vi "Launch UI.vi"(8 "error in (no error)":errorcluster, 11 "Test Application Controller in":refnum<class "Test Application Controller.lvclass">) -> (0 "error out":errorcluster, 3 "Test Application Controller out":refnum<class "Test Application Controller.lvclass">)   [LabVIEW 2017, in "Test Application Controller.lvlib" / "Test Application Controller.lvclass"]
uses:
  Test Application Controller.lvclass
  C:/Program Files (x86)/National Instruments/LabVIEW 2017/vi.lib/ActorFramework/Actor/Actor.lvclass
  User Interface/User Interface.lvclass
  Test Application Controller Messages/Start Test Msg/Start Test Msg.lvclass
  D:/Career/Tesla/LabVIEW_Interview_Problem/Tesla Test Application/User Interface Messages/Start Test Msg/Start Test Msg.lvclass
  Test Application Controller Messages/Close Application Msg/Close Application Msg.lvclass
  D:/Career/Tesla/LabVIEW_Interview_Problem/Tesla Test Application/User Interface Messages/Close Application Msg/Close Application Msg.lvclass
  Test Application Controller Messages/Stop Test Msg/Stop Test Msg.lvclass
  D:/Career/Tesla/LabVIEW_Interview_Problem/Tesla Test Application/User Interface Messages/Stop Test Msg/Stop Test Msg.lvclass
  Test Application Controller Messages/Generate Report Msg/Generate Report Msg.lvclass
  D:/Career/Tesla/LabVIEW_Interview_Problem/Tesla Test Application/User Interface Messages/Generate Report Msg/Generate Report Msg.lvclass
  User Interface/User Interface.lvclass/User Interface.ctl
  Test Application Controller.lvclass/Test Application Controller.ctl
  <vilib>/ActorFramework/Actor/Actor.lvclass
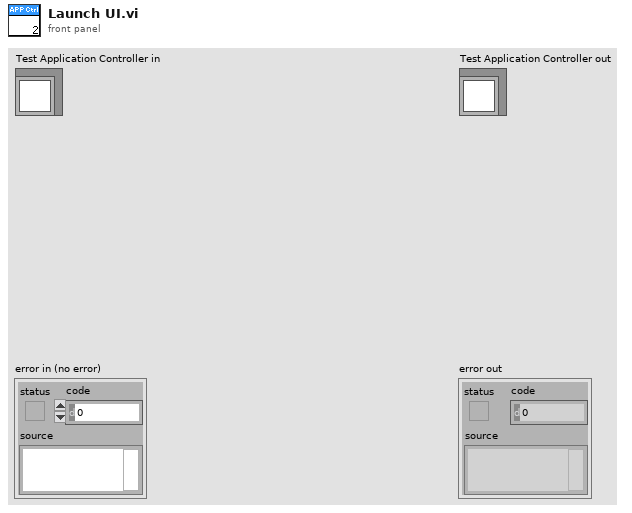
[diagram p1: front panel]
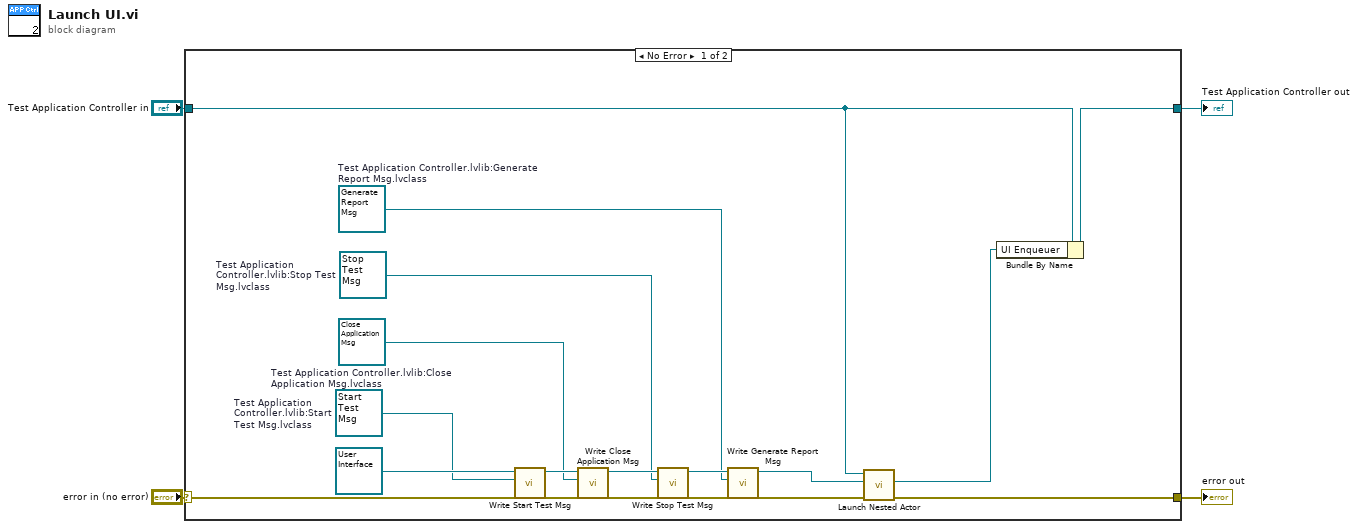
[diagram p0: block diagram]
diagram:
  n1 = case shown="No Error" "error in (no error)" {
    selector: "error in (no error)" -> [w18 w20]
    tunnel: [w17 w20] -> w3
    tunnel: [w11 w19] -> w1
    tunnel: "Test Application Controller in" -> [w15 w19]
    frame No Error {
      w5 = refnum<class "Generate Report Msg.lvclass"> refnum  # Test Application Controller.lvlib:Generate Report Msg.lvclass
      w8 = refnum<class "Stop Test Msg.lvclass"> refnum  # Test Application Controller.lvlib:Stop Test Msg.lvclass
      w12 = refnum<class "Close Application Msg.lvclass"> refnum  # Test Application Controller.lvlib:Close Application Msg.lvclass
      w14 = refnum<class "Start Test Msg.lvclass"> refnum  # Test Application Controller.lvlib:Start Test Msg.lvclass
      n2 = call "Write Start Test Msg.vi"("User Interface.lvlib:Start Test Msg.lvclass"=w14, "User Interface in"=refnum<class "User Interface.lvclass"> refnum ("User Interface.lvlib:User Interface.lvclass")) -> ("User Interface out"=w13:refnum<class "User Interface.lvclass">)  [unwired: 9 in]
      n3 = call "Write Close Application Msg.vi"("User Interface.lvlib:Close Application Msg.lvclass"=w12, "User Interface in"=w13) -> ("User Interface out"=w9:refnum<class "User Interface.lvclass">)  [unwired: 9 in]
      n4 = call "Write Stop Test Msg.vi"("User Interface.lvlib:Stop Test Msg.lvclass"=w8, "User Interface in"=w9) -> ("User Interface out"=w7:refnum<class "User Interface.lvclass">)  [unwired: 9 in]
      n5 = call "Write Generate Report Msg.vi"("User Interface.lvlib:Generate Report Msg.lvclass"=w5, "User Interface in"=w7) -> ("User Interface out"=w6:refnum<class "User Interface.lvclass">)  [unwired: 9 in]
      n6 = call <vilib>:"Launch Nested Actor.vi"("error in (no error)"=w18, "Nested Actor"=w6, "Caller Actor in"=w15) -> ("error out"=w17:errorcluster, "Nested Actor's Enqueuer"=w10:refnum<class "Message Enqueuer.lvclass">)  [unwired: 6 in, 1 out]
      n7 = Bundle By Name(cluster=w15, "UI Enqueuer"=w10) -> (w11:refnum<class "Test Application Controller.lvclass">)
    }
    frame Error {
    }
  }
  "error out" <- w3
  "Test Application Controller out" <- w1
